vi "day 15 task 1 even less memory neat.vi"() -> ()   [LabVIEW 2019]
uses:
  ea9792ab-c008-474f-a9ee-41b1ac887620.vi
panel:
  out "sorted array":cluster{"x":i32, "y":i32}[](array[cluster])
  out "size(s)":i32
  # "should be 26: don't include beacons!"
  # "0"
  # "Issue: 4,10 should not be there"
  # "0"
  # "10"
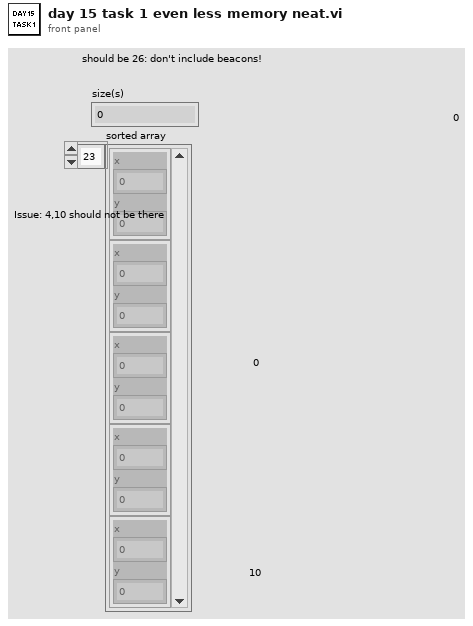
[diagram p1: front panel]
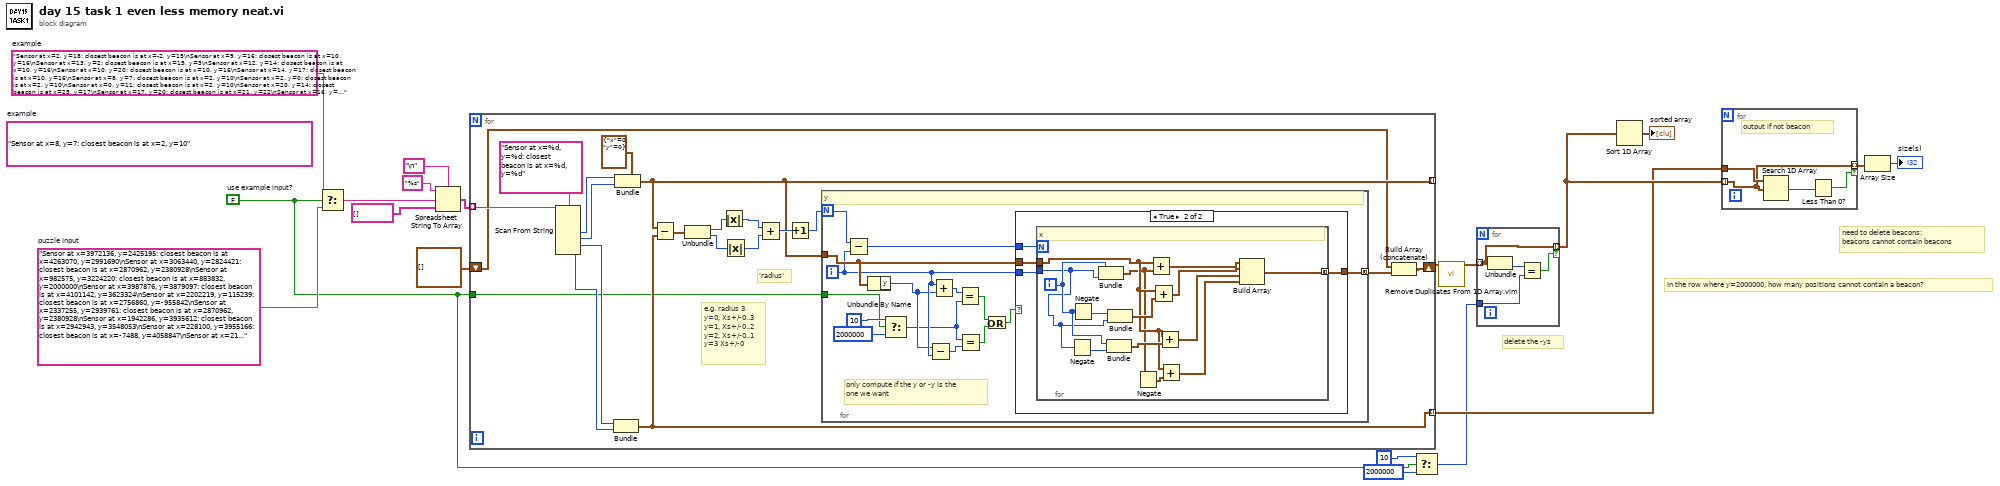
[diagram p0: block diagram]
diagram:
  w9 = "Sensor at x=2, y=18: closest beacon is at x=-2, y=15\nSensor at x=9, y=16: closest beacon is at x=10, y=16\nSensor at x=13, y=2: closest beacon is at x=15, y=3\nSensor at x=12, y=14: closest beacon is at x=10, y=16\nSensor at x=10, y=20: closest beacon is at x=10, y=16\nSensor at x=14, y=17: closest beacon is at x=10, y=16\nSensor at x=8, y=7: closest beacon is at x=2, y=10\nSensor at x=2, y=0: closest beacon is at x=2, y=10\nSensor at x=0, y=11: closest beacon is at x=2, y=10\nSensor at x=20, y=14: closest beacon is at x=25, y=17\nSensor at x=17, y=20: closest beacon is at x=21, y=22\nSensor at x=16, y=7: closest beacon is at x=15, y=3\nSensor at x=14, y=3: closest beacon is at x=15, y=3\nSensor at x=20, y=1: closest beacon is at x=15, y=3"  # example
  w1 = FALSE  # use example input?
  w16 = "Sensor at x=3972136, y=2425195: closest beacon is at x=4263070, y=2991690\nSensor at x=3063440, y=2824421: closest beacon is at x=2870962, y=2380928\nSensor at x=982575, y=3224220: closest beacon is at x=883832, y=2000000\nSensor at x=3987876, y=3879097: closest beacon is at x=4101142, y=3623324\nSensor at x=2202219, y=115239: closest beacon is at x=2756860, y=-955842\nSensor at x=2337255, y=2939761: closest beacon is at x=2870962, y=2380928\nSensor at x=1942286, y=3935612: closest beacon is at x=2942943, y=3548053\nSensor at x=228100, y=3955166: closest beacon is at x=-7488, y=4058847\nSensor at x=2114394, y=2368537: closest beacon is at x=2870962, y=2380928\nSensor at x=3658485, y=2855273: closest beacon is at x=4263070, y=2991690\nSensor at x=3731843, y=3995527: closest beacon is at x=4101142, y=3623324\nSensor at x=1311535, y=1294676: closest beacon is at x=883832, y=2000000\nSensor at x=3533617, y=3590533: closest beacon is at x=4101142, y=3623324\nSensor at x=341495, y=287725: closest beacon is at x=110643, y=-1160614\nSensor at x=1533864, y=2131620: closest beacon is at x=883832, y=2000000\nSensor at x=1179951, y=1876387: closest beacon is at x=883832, y=2000000\nSensor at x=3403590, y=1619877: closest beacon is at x=2870962, y=2380928\nSensor at x=2756782, y=3344622: closest beacon is at x=2942943, y=3548053\nSensor at x=14753, y=3818113: closest beacon is at x=-7488, y=4058847\nSensor at x=3808841, y=388411: closest beacon is at x=4559391, y=972750\nSensor at x=3129774, y=3401225: closest beacon is at x=2942943, y=3548053\nSensor at x=2710780, y=3978709: closest beacon is at x=2942943, y=3548053\nSensor at x=88084, y=2475915: closest beacon is at x=883832, y=2000000\nSensor at x=2503969, y=3564612: closest beacon is at x=2942943, y=3548053\nSensor at x=3954448, y=3360708: closest beacon is at x=4101142, y=3623324\nSensor at x=2724475, y=1736595: closest beacon is at x=2870962, y=2380928"  # puzzle input
  (unwired) "Sensor at x=8, y=7: closest beacon is at x=2, y=10"  # example
  # "delete the -ys"
  # "need to delete beacons:\nbeacons cannot contain beacons"
  # "In the row where y=2000000, how many positions cannot contain a beacon?"
  n1 = Select(t=w9, s=w1, f=w16) -> (s? t:f=w15:string)
  n2 = Spreadsheet String To Array(delimiter (Tab)="\n", format string="%s", spreadsheet string=w15, array type (2D Dbl)=string[] []) -> (array=w14:string[])
  n3 = for {
    tunnel: w14 -> [w39] mode=indexing
    tunnel: [w29] -> _ mode=indexing
    tunnel: [w28] -> w6 mode=indexing
    shift-right: [w21] -> w13
    shift-left: cluster{"x":i32, "y":i32}[] [] -> [w27]
    tunnel: w1 -> [w20]
    # "e.g. radius 3\ny=0, Xs+/-0..3\ny=1, Xs+/-0..2\ny=2, Xs+/-0..1\ny=3 Xs+/-0"
    # "'radius'"
    n4 = Scan From String(format string="Sensor at x=%d, y=%d: closest beacon is at x=%d, y=%d", input string=w39) -> (output 1=w33:i32, output 2=w35:i32, output 3=w36:i32, output 4=w34:i32)  [unwired: 6 in, 3 out]
    n5 = Bundle(w36, w34) -> (w28:cluster{i32, i32})  [unwired: 1 in]
    n6 = Bundle(cluster=cluster{"x":i32, "y":i32} {"x"=0, "y"=0}, "x"=w33, "y"=w35) -> (w29:cluster{"x":i32, "y":i32})
    n7 = Subtract(x=w29, y=w28) -> (x-y=w32:cluster{i32, i32})
    n8 = Unbundle(w32) -> (w24:i32, w22:i32)
    n9 = Absolute Value(x=w24) -> (abs(x)=w25:i32)
    n10 = Absolute Value(x=w22) -> (abs(x)=w23:i32)
    n11 = Add(x=w25, y=w23) -> (x+y=w31:i32)
    n12 = Increment(x=w31) -> (x+1=w26:i32)
    n13 = for {
      N: w26 -> [w53]
      tunnel: w29 -> [w51]
      tunnel: [w54] -> w30 mode=concatenating
      tunnel: w20 -> [w40]
      i -> [w49]
      # "only compute if the y or -y is the\none we want"
      # "y"
      n14 = Subtract(x=w53, y=w49) -> (x-y=w52:i32)
      n15 = Unbundle By Name(w51) -> ("y"=w48:i32)
      n16 = Select(t=10 ("y"), s=w40, f=2000000) -> (s? t:f=w41:i32)
      n17 = Subtract(x=w48, y=w49) -> (x-y=w47:i32)
      n18 = Add(x=w49, y=w48) -> (x+y=w50:i32)
      n19 = Equal?(x=w50, y=w41) -> (x = y?=w45:bool)
      n20 = Equal?(x=w41, y=w47) -> (x = y?=w46:bool)
      n21 = Or(x=w45, y=w46) -> (x .or. y?=w44:bool)
      n22 = case shown="True" w44 {
        tunnel: w51 -> [_ w58]
        tunnel: [_ w57] -> w54
        tunnel: w49 -> [_ w56]
        tunnel: w52 -> [_ w55]
        frame False {
        }
        frame True {
          n23 = for {
            N: w55 -> [_]
            tunnel: w56 -> [w65]
            tunnel: w58 -> [w63]
            tunnel: [w71] -> w57 mode=concatenating
            i -> [w66]
            # "x"
            n24 = Negate(x=w65) -> (-x=w67:i32)
            n25 = Negate(x=w66) -> (-x=w70:i32)
            n26 = Bundle(w66, w65) -> (w62:cluster{i32, i32})  [unwired: 1 in]
            n27 = Bundle(w66, w67) -> (w64:cluster{i32, i32})  [unwired: 1 in]
            n28 = Bundle(w70, w65) -> (w69:cluster{i32, i32})  [unwired: 1 in]
            n29 = Negate(x=w62) -> (-x=w61:cluster{i32, i32})
            n30 = Add(x=w63, y=w62) -> (x+y=w72:cluster{i32, i32})
            n31 = Add(x=w63, y=w69) -> (x+y=w68:cluster{i32, i32})
            n32 = Add(x=w63, y=w64) -> (x+y=w60:cluster{i32, i32})
            n33 = Add(x=w63, y=w61) -> (x+y=w59:cluster{i32, i32})
            n34 = Build Array(w72, w68, w60, w59) -> (w71:cluster{i32, i32}[])
          }
        }
      }
    }
    n35 = Build Array (concatenate)(w27, w30) -> (w21:cluster{"x":i32, "y":i32}[])
  }
  n36 = Select(t=10 ("y"), s=w1, f=2000000) -> (s? t:f=w2:i32)
  n37 = call "Remove Duplicates From 1D Array.vim"("array"=w13) -> ("array with duplicates removed"=w10:cluster{"x":i32, "y":i32}[])  [unwired: 10 in]
  n38 = for {
    tunnel: w10 -> [w74] mode=indexing
    tunnel: [w74] -> w7 mode=indexing if=w75
    tunnel: w2 -> [w73]
    n39 = Unbundle(w74) -> ("y"=w76:i32)  [unwired: 1 out]
    n40 = Equal?(x=w76, y=w73) -> (x = y?=w75:bool)
  }
  n41 = Sort 1D Array(array=w7) -> (sorted array=→"sorted array":cluster{"x":i32, "y":i32}[])
  n42 = for {
    tunnel: w7 -> [w77] mode=indexing
    tunnel: w6 -> [w78]
    tunnel: [w77] -> w5 mode=indexing if=w79
    # "output if not beacon"
    n43 = Search 1D Array(1D array=w78, element=w77) -> (index of element=w80:i32)  [unwired: 1 in]
    n44 = Less Than 0?(x=w80) -> (x < 0?=w79:bool)
  }
  n45 = Array Size(array=w5) -> (size(s)=→"size(s)":i32)
